vi "user process.vi"(8 "error in":errorcluster, 10 "Parameters to process":T2, 11 "user module in":refnum<class "user control module.lvclass">) -> (0 "error out":errorcluster, 2 "Results from processing":T1, 3 "user module out":refnum<class "user control module.lvclass">)   [LabVIEW 2014, in "user control module.lvclass"]
uses:
  user control module.lvclass
  parameter user data.ctl
  result user data.ctl
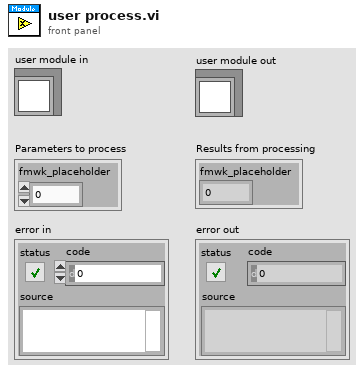
[diagram p1: front panel]
types:
  T1 = typedef "user control module.lvclass/result user data.ctl" = cluster{"fmwk_placeholder":sgl}
  T2 = typedef "user control module.lvclass/parameter user data.ctl" = cluster{"fmwk_placeholder":sgl}
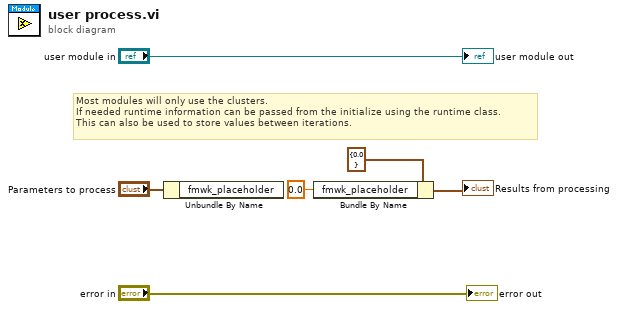
[diagram p0: block diagram]
diagram:
  # "Most modules will only use the clusters.\nIf needed runtime information can be passed from the initialize using the runtime class.\nThis can also be used to store values between iterations."
  n1 = Unbundle By Name("Parameters to process") -> ()  [unwired: 1 out]
  n2 = Bundle By Name(cluster=T1 {"fmwk_placeholder"=0.0} ("Results from processing"), "fmwk_placeholder"=sgl 0.0) -> (→"Results from processing":T1)
  "error out" <- "error in"
  "user module out" <- "user module in"
